vi "FilterRedPlane.vi"(2 "threshold":cluster{u8, u8}(slide)={0, 44} scale=0.0..255.0, 3 "Image in":T1 {"Dialogs" format="%.0b"}) -> (0 "image":picture, 1 "Image out":T1 {"Dialogs" format="%.0b"})   [LabVIEW 2024]
doc: "This VI allows a user to build a binary mask from red values between the threshold boundaries."
uses:
  <userlib>/ImageProcessing/QTLIB_2595_LV86/QT_Image.ctl
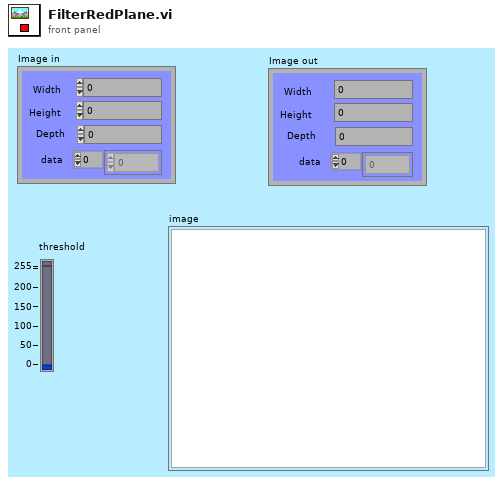
[diagram p1: front panel]
types:
  T1 = typedef "QT_Image.ctl" = cluster{"Width":i32, "Height":i32, "Depth":i32, "data":u8[], "Compressed data":u8[], "Color table":u32[], "Duration":i32, "Options":i32, "Timestamp":i32, "ID":i32, "Reserved":i32, "Dialogs":u32}
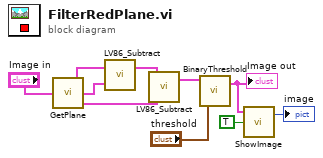
[diagram p0: block diagram]
diagram:
  n1 = call <userlib>:"GetPlane.vi"("Image In"="Image in") -> ("Blue Plane Out"=w6:T1, "Green Plane Out"=w8:T1, "Red Plane Out"=w9:T1)
  n2 = call <userlib>:"LV86_Subtract.vi"("Image 2"=w8, "Image"=w9) -> ("Image Out"=w7:T1)  [unwired: 1 in]
  n3 = call <userlib>:"LV86_Subtract.vi"("Image 2"=w6, "Image"=w7) -> ("Image Out"=w5:T1)  [unwired: 1 in]
  n4 = call <userlib>:"BinaryThreshold.vi"("threshold"="threshold", "Image In"=w5) -> ("Image Out"=w3:T1)  [unwired: 1 in]
  "Image out" <- w3
  n5 = call <userlib>:"ShowImage.vi"("Autoscale?"=TRUE, "Image"=w3) -> ("image"=→"image":picture)  [unwired: 1 in, 1 out]
